vi "Control Indicator Variable.vi"() -> ()   [LabVIEW 2010]
panel:
  in  "Control Indicator Array":dbl[](array[numeric])
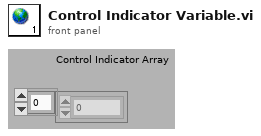
[diagram p1: front panel]
diagram:
